vi "Queue Self Alias Core.vi"(10 "Queue Mailbox":refnum<data-value>, 11 "jettl in":refnum<class "jettl.lvclass">) -> (2 "Self Alias":string, 3 "jettl out":refnum<class "jettl.lvclass">)   [LabVIEW 2021, in "jettl.lvlib" / "jettl.lvclass"]
uses:
  jettl.lvclass
  jettl.lvlib
  Queue Mailbox/Queue Mailbox.lvclass
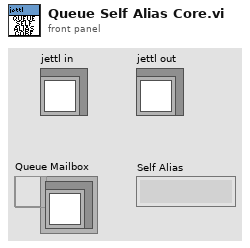
[diagram p1: front panel]
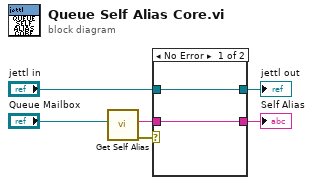
[diagram p0: block diagram]
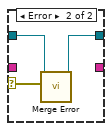
[diagram p2: hidden frame]
diagram:
  n1 = call "Get Self Alias.vi"("Queue Mailbox"="Queue Mailbox") -> ("error out"=w4:errorcluster, "Self Alias"=w1:string)  [unwired: 9 in]
  n2 = case shown="No Error" w4 {
    selector: w4 -> [_ w9]
    tunnel: [w8 w10] -> w6
    tunnel: "jettl in" -> [w8 w11]
    tunnel: [w7 _] -> w2
    tunnel: w1 -> [w7 _]
    frame No Error {
    }
    frame Error {
      n3 = call-dynamic "Merge Error.vi"("Error"=w9, "Merge Error in"=w11) -> ("Merge Error out"=w10:refnum<class "jettl.lvclass">)  [unwired: 9 in]
    }
  }
  "jettl out" <- w6
  "Self Alias" <- w2
